vi "Joystick.vi"(8 "Joystick error in":errorcluster) -> (0 "Joystick error out":errorcluster, 2 "Joystick":T1, 3 "Refnum out":refnum<k1>)   [LabVIEW 2016, in "ArgoBotLib.lvlib"]
uses:
  <vilib>/Utility/inputDevices.llb/joystickAcquire.vi
  ArgoBotLib.lvlib
panel:
  # "Joystick Button Config"
  # "This vi converts the joystick array to be named the same as the Xbox controller buttons  and scalled the same as a FRC robot"
  # "Inputs"
  # "Outputs"
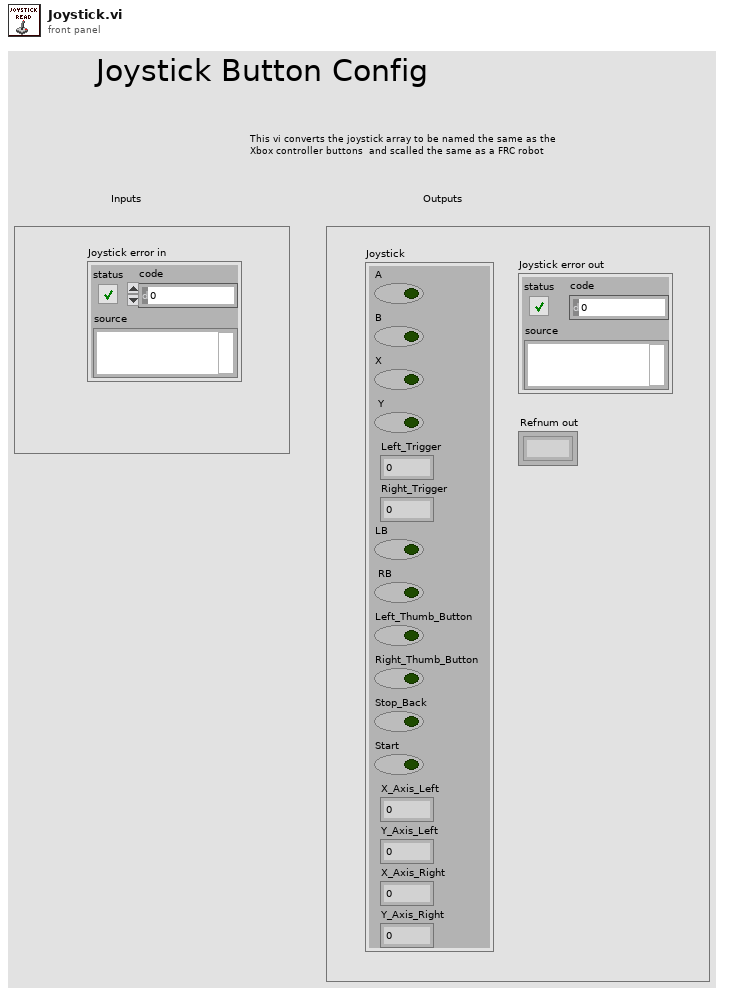
[diagram p1: front panel]
types:
  T1 = cluster{"A":bool, "B":bool, "X":bool, " Y":bool, "Left_Trigger":dbl, "Right_Trigger ":dbl, "LB":bool, " RB":bool, "Left_Thumb_Button":bool, "Right_Thumb_Button":bool, "Stop_Back":bool, "Start":bool, "X_Axis_Left":dbl, "Y_Axis_Left":dbl, "X_Axis_Right":dbl, "Y_Axis_Right":dbl}
  T2 = cluster{"X axis":i32, "Y axis":i32, "Z axis":i32, "X axis rotation":i32, "Y axis rotation":i32, "Z axis rotation":i32, "U axis":i32, "V axis":i32}
  T3 = cluster{"button 1":bool, "button 2":bool, "button 3":bool, "button 4":bool, "button 5":bool, "button 6":bool, "button 7":bool, "button 8":bool, "button 9":bool, "button 10":bool, "button 11":bool, "button 12":bool, "button 13":bool, "button 14":bool, "button 15":bool, "button 16":bool, "button 17":bool, "button 18":bool, "button 19":bool, "button 20":bool, "button 21":bool, "button 22":bool, "button 23":bool, "button 24":bool, "button 25":bool, "button 26":bool, "button 27":bool, "button 28":bool, "button 29":bool, "button 30":bool, "button 31":bool, "button 32":bool}
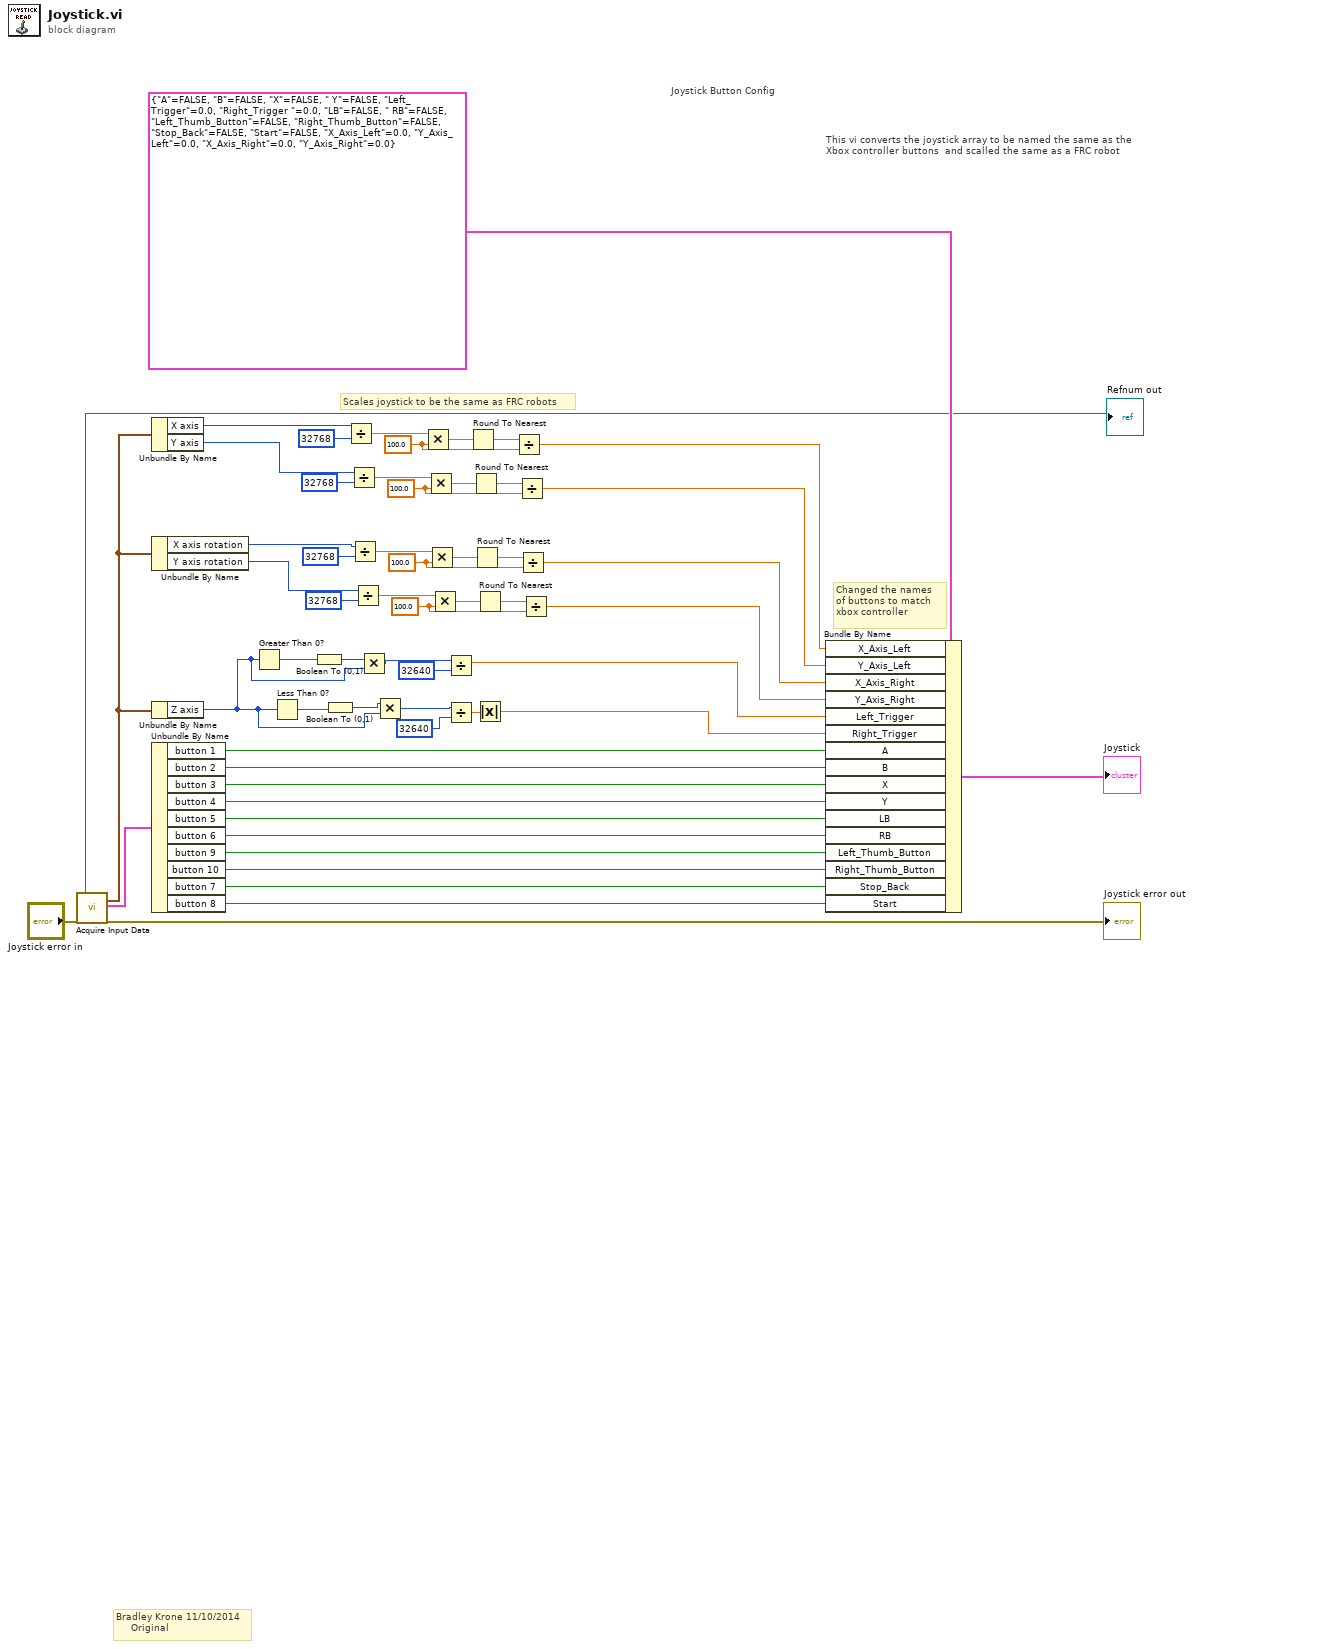
[diagram p0: block diagram]
diagram:
  w50 = 100.0 ("y")
  w45 = 100.0 ("y")
  w39 = 100.0 ("y")
  w34 = 100.0 ("y")
  # "Changed the names \nof buttons to match \nxbox controller"
  # "Scales joystick to be the same as FRC robots"
  # "This vi converts the joystick array to be named the same as the Xbox controller buttons  and scalled the same as a FRC robot"
  # "Joystick Button Config"
  # "Bradley Krone 11/10/2014\n     Original"
  n1 = call-poly <vilib>:"Acquire Input Data.vi"("error in (no error)"="Joystick error in") -> ("device ID"=→"Refnum out":refnum<k1>, "axis info"=w28:T2, "button info"=w3:T3, "error out"=→"Joystick error out":errorcluster)  [unwired: 1 in, 14 out]
  n2 = Unbundle By Name(w28) -> ("X axis"=w29:i32, "Y axis"=w40:i32)
  n3 = Unbundle By Name(w28) -> ("X axis rotation"=w51:i32, "Y axis rotation"=w52:i32)
  n4 = Unbundle By Name(w28) -> ("Z axis"=w24:i32)
  n5 = Unbundle By Name(w3) -> ("button 1"=w5:bool, "button 2"=w6:bool, "button 3"=w7:bool, "button 4"=w8:bool, "button 5"=w9:bool, "button 6"=w10:bool, "button 9"=w11:bool, "button 10"=w12:bool, "button 7"=w13:bool, "button 8"=w14:bool)
  n6 = Greater Than 0?(x=w24) -> (x > 0?=w17:bool)
  n7 = Less Than 0?(x=w24) -> (x < 0?=w22:bool)
  n8 = Boolean To (0,1)(Boolean=w17) -> (0, 1=w16:i16)
  n9 = Boolean To (0,1)(Boolean=w22) -> (0, 1=w23:i16)
  n10 = Divide(x=w29, y=32768) -> (x/y=w31:dbl)
  n11 = Divide(x=w40, y=32768) -> (x/y=w36:dbl)
  n12 = Divide(x=w51, y=32768) -> (x/y=w42:dbl)
  n13 = Divide(x=w52, y=32768) -> (x/y=w47:dbl)
  n14 = Multiply(x=w16, y=w24) -> (x*y=w19:i32)
  n15 = Multiply(x=w23, y=w24) -> (x*y=w25:i32)
  n16 = Multiply(x=w31, y=w34) -> (x*y=w32:dbl)
  n17 = Multiply(x=w36, y=w39) -> (x*y=w37:dbl)
  n18 = Multiply(x=w42, y=w45) -> (x*y=w43:dbl)
  n19 = Multiply(x=w47, y=w50) -> (x*y=w48:dbl)
  n20 = Divide(x=w19, y=32640) -> (x/y=w18:dbl)
  n21 = Divide(x=w25, y=32640) -> (x/y=w26:dbl)
  n22 = Round To Nearest(number=w32) -> (nearest integer value=w33:dbl)
  n23 = Round To Nearest(number=w37) -> (nearest integer value=w38:dbl)
  n24 = Round To Nearest(number=w43) -> (nearest integer value=w44:dbl)
  n25 = Round To Nearest(number=w48) -> (nearest integer value=w49:dbl)
  n26 = Absolute Value(x=w26) -> (abs(x)=w27:dbl)
  n27 = Divide(x=w33, y=w34) -> (x/y=w53:dbl)
  n28 = Divide(x=w38, y=w39) -> (x/y=w54:dbl)
  n29 = Divide(x=w44, y=w45) -> (x/y=w55:dbl)
  n30 = Divide(x=w49, y=w50) -> (x/y=w56:dbl)
  n31 = Bundle By Name(cluster=T1 {"A"=FALSE, "B"=FALSE, "X"=FALSE, " Y"=FALSE, "Left_Trigger"=0.0, "Right_Trigger "=0.0, "LB"=FALSE, " RB"=FALSE, "Left_Thumb_Button"=FALSE, "Right_Thumb_Button"=FALSE, "Stop_Back"=FALSE, "Start"=FALSE, "X_Axis_Left"=0.0, "Y_Axis_Left"=0.0, "X_Axis_Right"=0.0, "Y_Axis_Right"=0.0}, "X_Axis_Left"=w53, "Y_Axis_Left"=w54, "X_Axis_Right"=w55, "Y_Axis_Right"=w56, "Left_Trigger"=w18, "Right_Trigger"=w27, "A"=w5, "B"=w6, "X"=w7, "Y"=w8, "LB"=w9, "RB"=w10, "Left_Thumb_Button"=w11, "Right_Thumb_Button"=w12, "Stop_Back"=w13, "Start"=w14) -> (→"Joystick":T1)
